vi "Create Clean Task.vi"(6 "Task Name":string, 8 "error in (no error)":errorcluster) -> (0 "error out":errorcluster, 3 "task out":refnum<k21>)   [LabVIEW 2019, in "4300.lvlib" / "4300.lvclass"]
uses:
  4300.lvclass
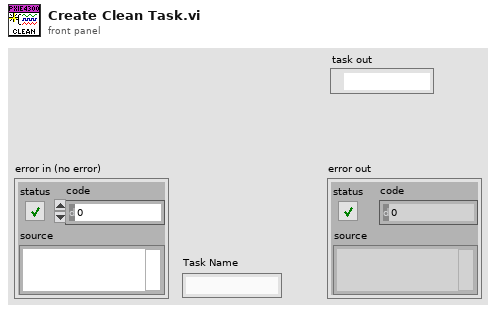
[diagram p1: front panel]
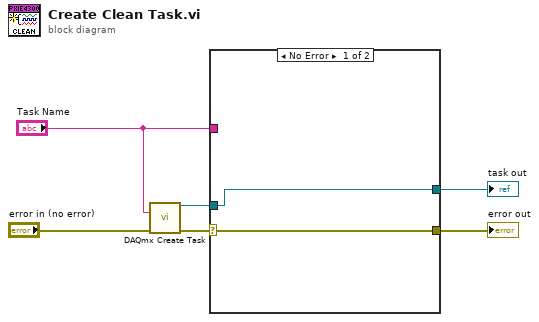
[diagram p0: block diagram]
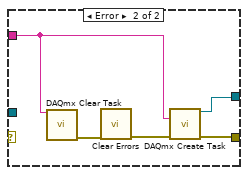
[diagram p2: hidden frame]
diagram:
  n1 = call <vilib>:"DAQmx Create Task.vi"("task to copy"="Task Name", "error in"="error in (no error)") -> ("task out"=w3:refnum<k21>, "error out"=w5:errorcluster)  [unwired: 12 in]
  n2 = case shown="No Error" w5 {
    selector: w5 -> [w8 _]
    tunnel: [w8 w10] -> w4
    tunnel: w3 -> [w7 _]
    tunnel: "Task Name" -> [_ w11]
    tunnel: [w7 w9] -> w1
    frame No Error {
    }
    frame Error {
      n3 = call <vilib>:"DAQmx Clear Task.vi"("task in"=w11) -> ("error out"=w13:errorcluster)  [unwired: 14 in]
      n4 = call <vilib>:"Clear Errors.vi"("error in (no error)"=w13) -> ("error out"=w12:errorcluster)  [unwired: 5 in, 1 out]
      n5 = call <vilib>:"DAQmx Create Task.vi"("task to copy"=w11, "error in"=w12) -> ("task out"=w9:refnum<k21>, "error out"=w10:errorcluster)  [unwired: 12 in]
    }
  }
  "error out" <- w4
  "task out" <- w1
